vi "DSF.Engine.Transceiver Thread.Get Transfer Groups.vi"(11 "Transceiver Thread in":refnum<class "DSF.Engine.Transceiver Thread.lvclass">) -> (2 "Transfer Groups":refnum<class "DSF.Engine.Transfer Group.lvclass">[](array[class]), 3 "Transceiver Thread out":refnum<class "DSF.Engine.Transceiver Thread.lvclass">)   [LabVIEW 2017, in "Data Sharing Framework Engine.lvlib" / "DSF.Engine.Transceiver Thread.lvclass"]
uses:
  DSF.Engine.Transceiver Thread.lvclass
  Transfer/DSF.Engine.Transfer Group.lvclass
  DSF.Engine.Transceiver Thread.lvclass/DSF.Engine.Transceiver Thread.ctl
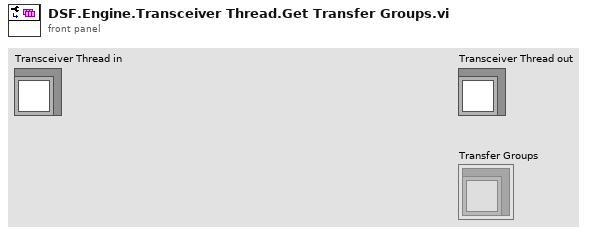
[diagram p1: front panel]
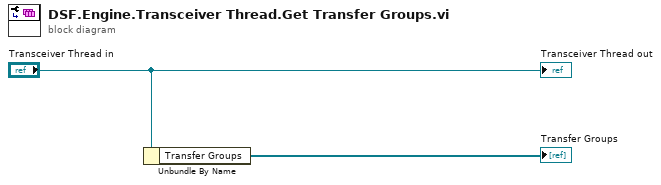
[diagram p0: block diagram]
diagram:
  n1 = Unbundle By Name("Transceiver Thread in") -> ("Transfer Groups"=→"Transfer Groups":refnum<class "DSF.Engine.Transfer Group.lvclass">[])
  "Transceiver Thread out" <- "Transceiver Thread in"
